vi "Tree Strings.vi"(8 "error in (no error)":errorcluster, 11 "Valve Item in":refnum<class "Valve Item.lvclass">) -> (0 "error out":errorcluster, 1 "Child Text":string[](array[string]), 2 "Left Cell String":string, 3 "Valve Item out":refnum<class "Valve Item.lvclass">, 5 "Child Tag":string)   [LabVIEW 2020, in "BetterDragAndDropDemo.lvlib" / "Valve Item.lvclass"]
uses:
  Valve Item.lvclass
  Valve Item.lvclass/Valve Item.ctl
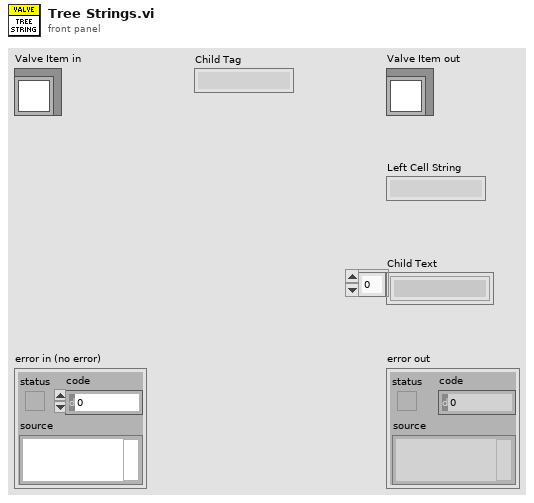
[diagram p1: front panel]
types:
  T1 = typedef "BetterDragAndDropDemo.lvlib/Valve Item.lvclass/valve color.ctl" = enum16{"black", "red"}
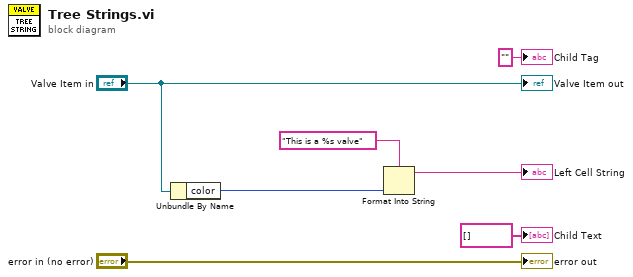
[diagram p0: block diagram]
diagram:
  n1 = Unbundle By Name("Valve Item in") -> ("color"=w3:T1)
  n2 = Format Into String(format string="This is a %s valve", w3) -> (resulting string=→"Left Cell String":string)  [unwired: 2 in, 1 out]
  "error out" <- "error in (no error)"
  "Valve Item out" <- "Valve Item in"
  "Child Text" <- string[] [] ("Child Text")
  "Child Tag" <- "" ("Child Tag")
